vi "ADC_range.vi"(4 "Channels & Spans":T1={"high limit (10V)"=10.0, "low limit (-10V)"=-10.0, "Ch No"=0, "Var name"="", "Use Latest Calib"=FALSE} {"low limit (-10V)" format="%.3f"; "high limit (10V)" format="%.3f"}) -> (0 "Range Code":i32, 1 "MaxABS( Voltage)":dbl format="%.2f")   [LabVIEW 2010]
uses:
  Controls/Ch_and_Spans.ctl
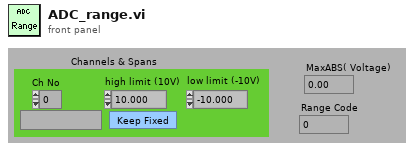
[diagram p1: front panel]
types:
  T1 = typedef "Ch_and_Spans.ctl" = cluster{"high limit (10V)":sgl, "low limit (-10V)":sgl, "Ch No":i16, "Var name":string, "Use Latest Calib":bool}
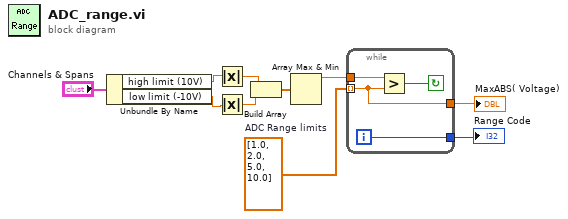
[diagram p0: block diagram]
diagram:
  w5 = dbl[] [1.0, 2.0, 5.0, 10.0]  # ADC Range limits
  n1 = Unbundle By Name ("Find absolute maximum voltage reqd for each channel")("Channels & Spans") -> ("high limit (10V)"=w8:sgl, "low limit (-10V)"=w9:sgl)
  n2 = Absolute Value(x=w8) -> (abs(x)=w7:sgl)
  n3 = Absolute Value(x=w9) -> (abs(x)=w6:sgl)
  n4 = Build Array(w7, w6) -> (w2:sgl[])
  n5 = Array Max & Min(array=w2) -> (max value=w3:sgl)  [unwired: 3 out]
  n6 = while {
    tunnel: [w11] -> w1
    tunnel: [w12] -> w4
    tunnel: w5 -> [w12] mode=indexing
    tunnel: w3 -> [w14]
    i -> [w11]
    stop <- w13 continue-if-true
    n7 = Greater?(x=w14, y=w12) -> (0:w13:bool)
  }
  "MaxABS( Voltage)" <- w4
  "Range Code" <- w1
